vi "start.vi"(8 "error in (no error)":errorcluster, 11 "Model in":refnum<class "Model.lvclass">) -> (0 "error out":errorcluster, 3 "Model out":refnum<class "Model.lvclass">)   [LabVIEW 2015, in "Model.lvclass"]
uses:
  Model.lvclass
  Model.lvclass/Model.ctl
  <userlib>/Common/ILC/ILC/ILC.lvclass/ILC.ctl
  <userlib>/Common/ILC/ILC/ILC.lvclass
  ApplicationElements/SystemController/SystemController.lvclass
  <userlib>/Common/Devices/DistanceGauge/DistanceGauge/DistanceGauge.lvclass
  <userlib>/Common/Devices/ForceSensorCalculator/ForceSensorCalculator/ForceSensorCalculator.lvclass
  <userlib>/Common/Devices/PressureValve/PressureValve/PressureValve.lvclass
  ApplicationElements/StiffnessCalculator/StiffnessCalculator.lvclass
  ApplicationElements/PreconditioningMonitor/PreconditioningMonitor.lvclass
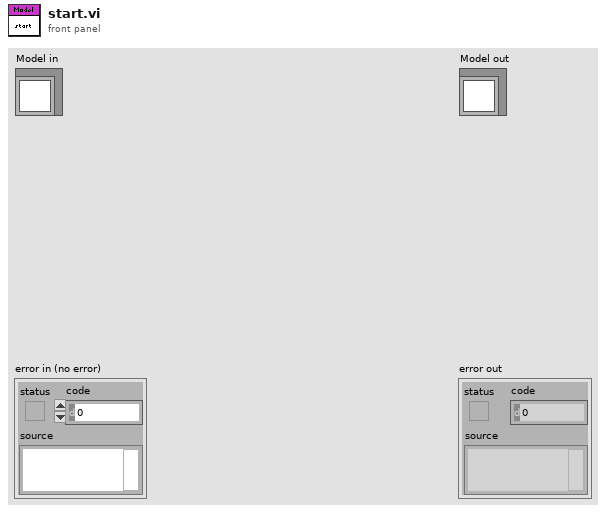
[diagram p1: front panel]
types:
  T1 = typedef "ILCCommon.lvlib/ILCConfiguration.lvlib/ILCADC.ctl" = cluster{"Input Channels":T2, "Scan Rate (Hz) ":T3, "PGA Gain Coefficient":u8, "Reference Voltage Vref":dbl[unit], "Nominal Input Range in Counts":u32, "Preamplifier Gain":u8, "Conversion Settling Cycles":u16}
  T2 = typedef "ILCCommon.lvlib/ILCConfiguration.lvlib/InputChannels.ctl" = enum16{"Channel 0", "3 Channels", "5 Channels"}
  T3 = typedef "ILCCommon.lvlib/ILCConfiguration.lvlib/ScanRate_Hz_MultichannelOptions.ctl" = enum16{"50", "60", "100", "120", "200", "240", "300", "400", "480", "600", "1200", "2400", "4800"}
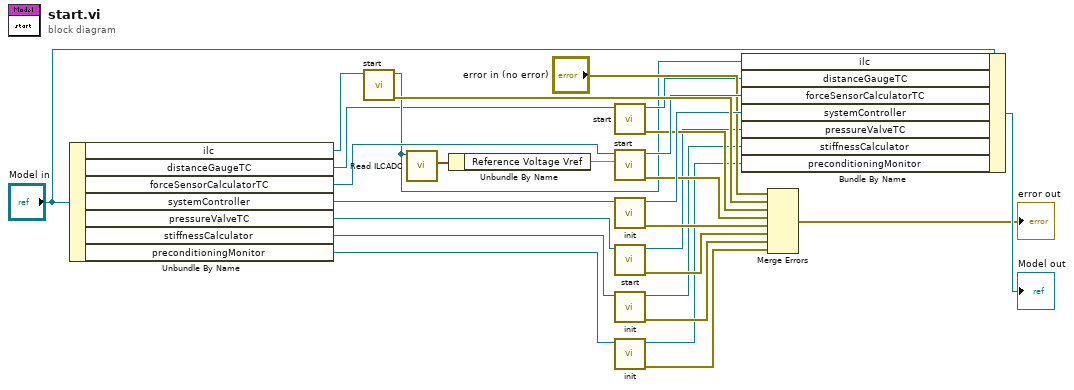
[diagram p0: block diagram]
diagram:
  n1 = Unbundle By Name("Model in") -> ("ilc"=w25:refnum<class "ILC.lvclass">, "distanceGaugeTC"=w10:refnum<class "DistanceGaugeTC.lvclass">, "forceSensorCalculatorTC"=w22:refnum<class "ForceSensorCalculatorTC.lvclass">, "systemController"=w20:refnum<class "SystemController.lvclass">, "pressureValveTC"=w9:refnum<class "PressureValveTC.lvclass">, "stiffnessCalculator"=w6:refnum<class "StiffnessCalculator.lvclass">, "preconditioningMonitor"=w3:refnum<class "PreconditioningMonitor.lvclass">)
  n2 = call <userlib>:"start.vi"("ILC in"=w25) -> ("error out"=w24:errorcluster, "ILC out"=w12:refnum<class "ILC.lvclass">)  [unwired: 9 in]
  n3 = call <userlib>:"Read ILCADC.vi"("ILC in"=w12) -> ("ILC ADC"=w13:T1)  [unwired: 9 in, 1 out]
  n4 = Unbundle By Name(w13) -> ("Reference Voltage Vref"=w11:dbl[unit])
  n5 = call <userlib>:"start.vi"("DistanceGauge in"=w10) -> ("error out"=w14:errorcluster, "DistanceGauge out"=w15:refnum<class "DistanceGaugeTC.lvclass">)  [unwired: 9 in]
  n6 = call <userlib>:"start.vi"("Reference Voltage Vref"=w11, "ForceSensor in"=w22) -> ("error out"=w17:errorcluster, "ForceSensor out"=w21:refnum<class "ForceSensorCalculatorTC.lvclass">)  [unwired: 8 in]
  n7 = call "init.vi"("SystemController in"=w20) -> ("error out"=w16:errorcluster, "SystemController out"=w19:refnum<class "SystemController.lvclass">)  [unwired: 9 in]
  n8 = call <userlib>:"start.vi"("PressureValve in"=w9) -> ("error out"=w7:errorcluster, "PressureValve out"=w8:refnum<class "PressureValveTC.lvclass">)  [unwired: 9 in]
  n9 = call "init.vi"("StiffnessCalculator in"=w6) -> ("error out"=w4:errorcluster, "StiffnessCalculator out"=w5:refnum<class "StiffnessCalculator.lvclass">)  [unwired: 9 in]
  n10 = call "init.vi"("PreconditioningMonitor in"=w3) -> ("error out"=w1:errorcluster, "PreconditioningMonitor out"=w2:refnum<class "PreconditioningMonitor.lvclass">)  [unwired: 9 in]
  n11 = Bundle By Name(cluster="Model in", "ilc"=w12, "distanceGaugeTC"=w15, "forceSensorCalculatorTC"=w21, "systemController"=w19, "pressureValveTC"=w8, "stiffnessCalculator"=w5, "preconditioningMonitor"=w2) -> (→"Model out":refnum<class "Model.lvclass">)
  n12 = Merge Errors("error in (no error)", w24, w14, w17, w16, w7, w4, w1) -> (→"error out":errorcluster)
